vi "Convert Error to Warning.vi"(2 "Error In":errorcluster) -> (7 "no Error Out":errorcluster)   [LabVIEW 2021]
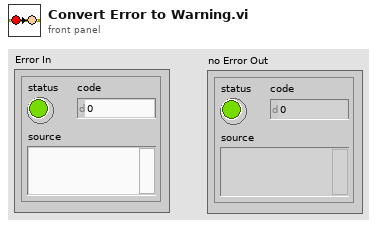
[diagram p1: front panel]
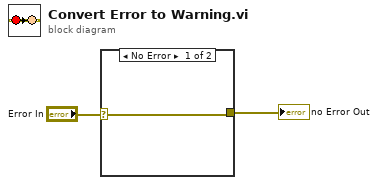
[diagram p0: block diagram]
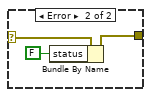
[diagram p2: hidden frame]
diagram:
  n1 = case shown="No Error" "Error In" {
    selector: "Error In" -> [w3 w6]
    tunnel: [w3 w5] -> w1
    frame No Error {
    }
    frame Error {
      n2 = Bundle By Name(cluster=w6, "status"=FALSE) -> (w5:errorcluster)
    }
  }
  "no Error Out" <- w1
